vi "Check Forward Collision.vi"(7 "Decrement Future? (F) in":bool, 11 "AI Manager in":refnum<class "AI Manager.lvclass">) -> (1 "Velocity out":T1, 2 "Collision coordinate out":T1, 4 "Vector direction out":cluster{dbl, dbl}, 5 "Collision?":bool)   [LabVIEW 2024, in "AI Manager.lvclass"]
doc: "MIT Licence\nCopyright (c) 2024 David Grollier"
uses:
  AI Manager.lvclass
  Type Def/Velocity.ctl
  AI Manager.lvclass/AI Manager.ctl
  Game Componants/Game Componants.lvclass/Game Componants.ctl
  Game Componants/Game Board Component/Movable/Movable.lvclass/Movable.ctl
  Game Componants/Game Board Component/Movable/Flying Saucer/Flying Saucer.lvclass/Flying Saucer.ctl
  <vilib>/Analysis/_algsub.llb/Vector Norm.vi
  <vilib>/Analysis/_algsub.llb/Real Vector Norm.vi
  Game Componants/Game Board Component/Movable/Flying Saucer/Flying Saucer.lvclass
  Game Componants/Game Board Component/Movable/Movable.lvclass
  Utils/Utils.lvlib
  Game Componants/Game Componants.lvclass
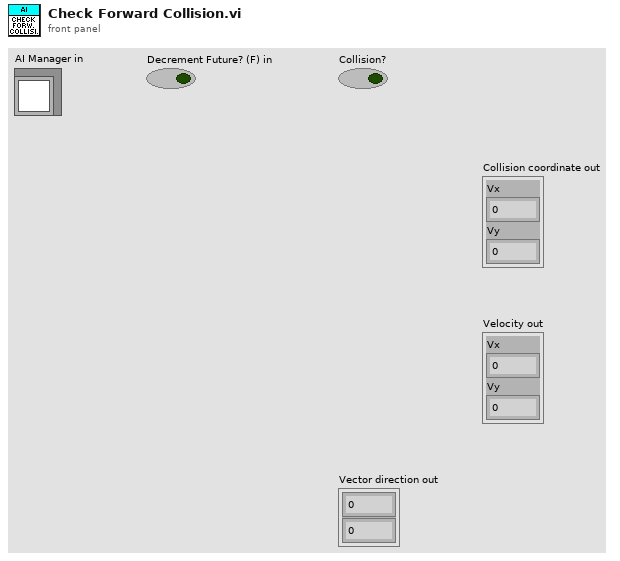
[diagram p1: front panel]
types:
  T1 = typedef "Velocity.ctl" = cluster{"Vx":dbl, "Vy":dbl}
  T2 = typedef "Coordinates.ctl" = cluster{"x":dbl, "y":dbl}
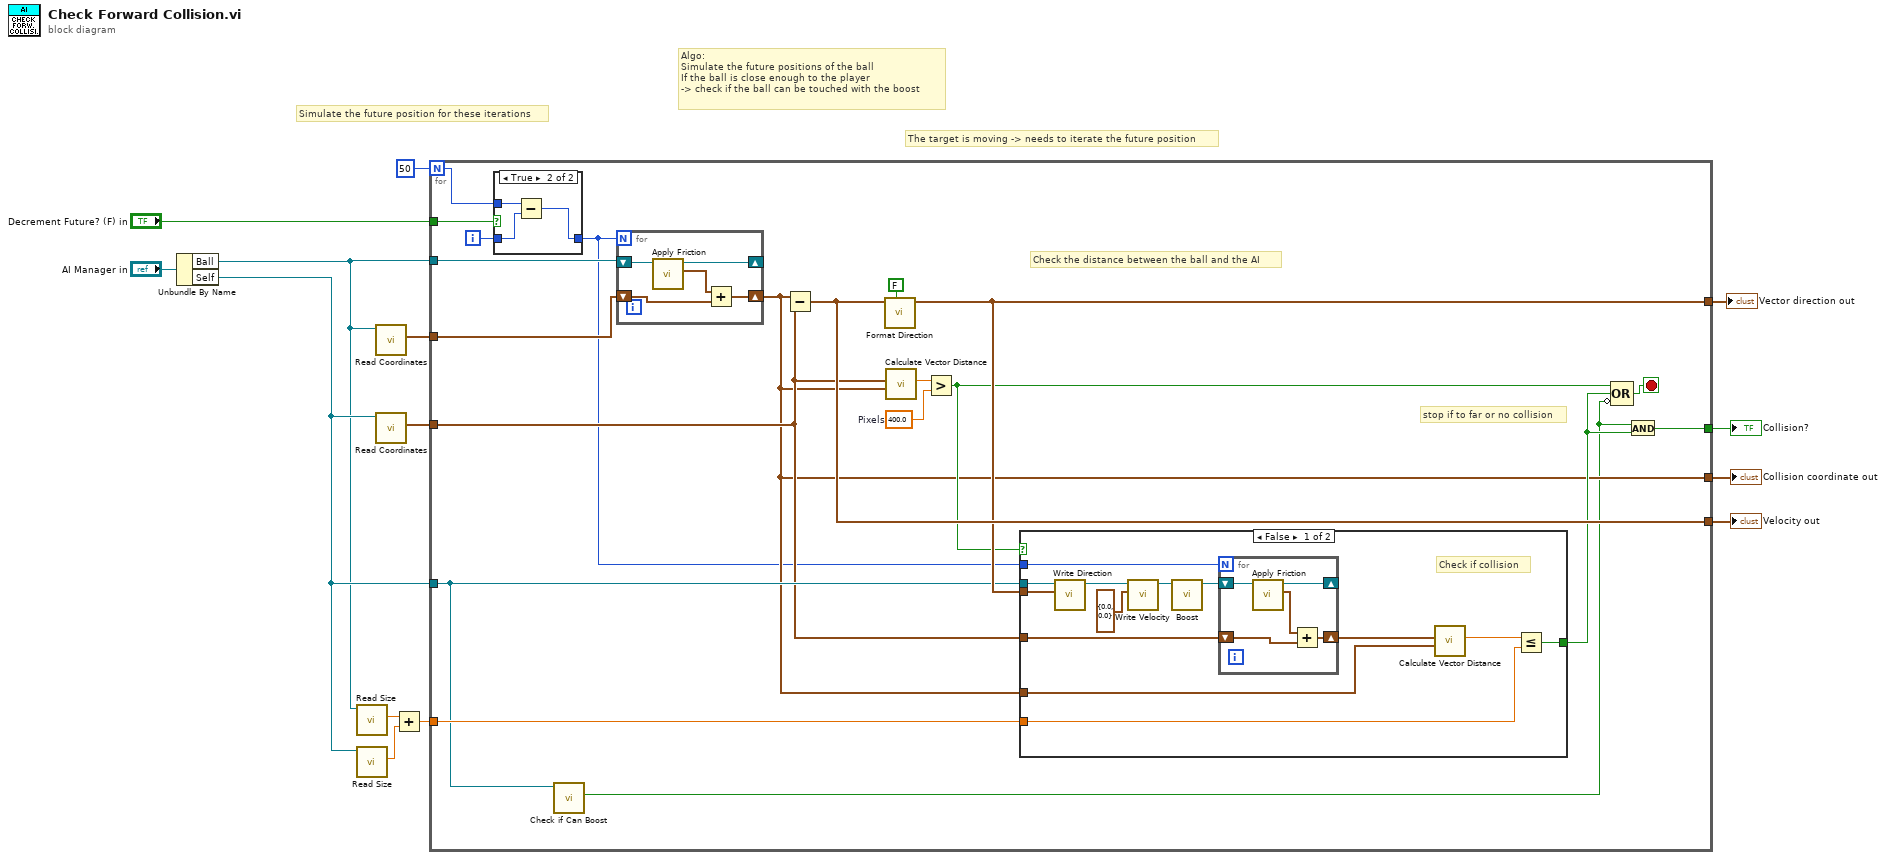
[diagram p0: block diagram]
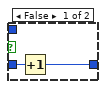
[diagram p2: hidden frame]
diagram:
  # "Algo:\nSimulate the future positions of the ball\nIf the ball is close enough to the player\n-> check if the ball can be touched with the boost"
  # "The target is moving -> needs to iterate the future position"
  # "Simulate the future position for these iterations"
  n1 = Unbundle By Name("AI Manager in") -> ("Ball"=w2:refnum<class "Movable.lvclass">, "Self"=w3:refnum<class "Flying Saucer.lvclass">)
  n2 = call "Read Size.vi"("Movable in"=w2) -> ("Size"=w9:dbl)  [unwired: 10 in]
  n3 = call "Read Size.vi"("Movable in"=w3) -> ("Size"=w10:dbl)  [unwired: 10 in]
  n4 = call "Read Coordinates.vi"("Game Componants in"=w2) -> ("Coordinates"=w12:T2)  [unwired: 10 in]
  n5 = call "Read Coordinates.vi"("Game Componants in"=w3) -> ("Coordinates"=w13:T2)  [unwired: 10 in]
  n6 = Add(x=w9, y=w10) -> (x+y=w11:dbl)
  n7 = for {
    N: 50 -> [w15]
    tunnel: [w23] -> w5
    tunnel: [w32] -> w6
    tunnel: w2 -> [w30]
    tunnel: [w21] -> w7
    tunnel: w3 -> [w28]
    tunnel: [w31] -> w8
    tunnel: w11 -> [w29]
    tunnel: w12 -> [w25]
    tunnel: w13 -> [w22]
    tunnel: "Decrement Future? (F) in" -> [w18]
    i -> [w17]
    stop <- w27 stop-if-true
    w33 = 400.0  # Pixels
    # "Check the distance between the ball and the AI"
    # "stop if to far or no collision"
    n8 = case shown="True" w18 {
      tunnel: w17 -> [w36 w38]
      tunnel: [w35 w37] -> w16
      tunnel: w15 -> [_ w39]
      frame False {
        n9 = Increment(x=w36) -> (x+1=w35:i32)
      }
      frame True {
        n10 = Subtract(x=w39, y=w38) -> (x-y=w37:i32)
      }
    }
    n11 = call "Check if Can Boost.vi"("Flying Saucer in"=w28) -> ("Can Boost?"=w19:bool)  [unwired: 10 in]
    n12 = for {
      N: w16 -> [_]
      shift-right: [w61] -> _
      shift-left: w30 -> [w62]
      shift-right: [w59] -> w21
      shift-left: w25 -> [w58]
      n13 = call "Apply Friction.vi"("Movable in"=w62) -> ("Velocity out"=w60:T1, "Movable out"=w61:refnum<class "Movable.lvclass">)  [unwired: 9 in]
      n14 = Add(x=w60, y=w58) -> (x+y=w59:T1)
    }
    n15 = Subtract(x=w21, y=w22) -> (x-y=w32:T1)
    n16 = call "Format Direction.vi"("Xbox Controller (T)"=FALSE ("Analog Stick? (T)"), "Direction in"=w32) -> ("Formated Direction out"=w31:cluster{dbl, dbl})  [unwired: 9 in]
    n17 = call "Calculate Vector Distance.vi"("V2"=w21, "V1"=w22) -> ("Distance out"=w20:dbl)  [unwired: 9 in]
    n18 = Greater?(x=w20, y=w33) -> (0:w26:bool)
    n19 = case shown="False" w26 {
      tunnel: w31 -> [w50 _]
      tunnel: w21 -> [w42 _]
      tunnel: w22 -> [w45 _]
      tunnel: w29 -> [w44 _]
      tunnel: w28 -> [w47 _]
      tunnel: [w43 _] -> w24
      tunnel: w16 -> [w46 _]
      frame False {
        # "Check if collision"
        n20 = call "Write Direction.vi"("Velocity"=w50, "Flying Saucer in"=w47) -> ("Flying Saucer out"=w49:refnum<class "Flying Saucer.lvclass">)  [unwired: 9 in]
        n21 = call "Write Velocity.vi"("Velocity"=T1 {"Vx"=0.0, "Vy"=0.0}, "Movable in"=w49) -> ("Movable out"=w52:refnum<class "Flying Saucer.lvclass">)  [unwired: 9 in]
        n22 = call "Boost.vi"("Flying Saucer in"=w52) -> ("Flying Saucer out"=w48:refnum<class "Flying Saucer.lvclass">)  [unwired: 10 in]
        n23 = for {
          N: w46 -> [_]
          shift-right: [w56] -> _
          shift-left: w48 -> [w57]
          shift-right: [w53] -> w41
          shift-left: w45 -> [w55]
          n24 = call "Apply Friction.vi"("Movable in"=w57) -> ("Velocity out"=w54:T1, "Movable out"=w56:refnum<class "Flying Saucer.lvclass">)  [unwired: 9 in]
          n25 = Add(x=w54, y=w55) -> (x+y=w53:T1)
        }
        n26 = call "Calculate Vector Distance.vi"("V2"=w42, "V1"=w41) -> ("Distance out"=w40:dbl)  [unwired: 9 in]
        n27 = Less Or Equal?(x=w40, y=w44) -> (x <= y?=w43:bool)
      }
      frame True {
      }
    }
    n28 = Compound Arithmetic op=OR(w26, w24, invert w19) -> (w27:bool)
    n29 = And(x=w19, y=w24) -> (x .and. y?=w23:bool)
  }
  "Vector direction out" <- w8
  "Collision coordinate out" <- w7
  "Velocity out" <- w6
  "Collision?" <- w5
